vi "Cartesian_to_polar.vi"(2 "Z-Axis (T)":dbl format="%#_13g", 3 "Y-Axis (T)":dbl format="%#_13g") -> (0 "phi (deg)":dbl min=0.0 format="%.3f", 1 "Radial (r) Field (T)":dbl min=0.0 format="%.3f")   [LabVIEW 2018]
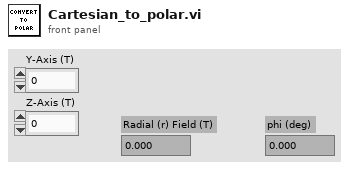
[diagram p1: front panel]
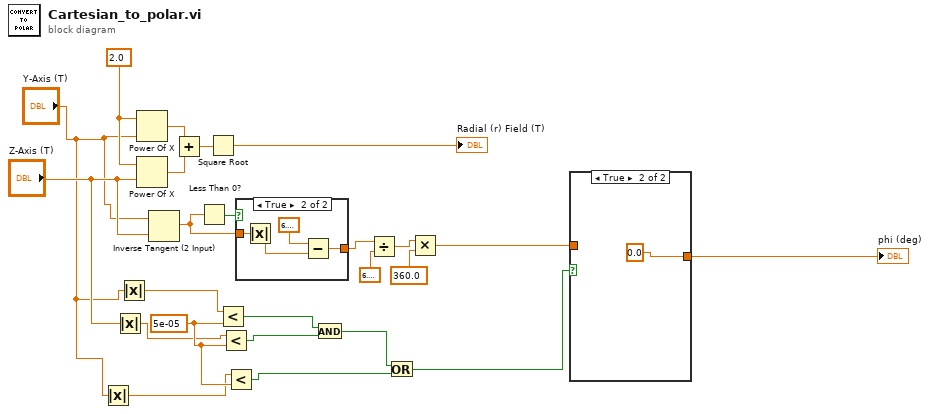
[diagram p0: block diagram]
diagram:
  w7 = 5e-05 ("y")
  w24 = 2.0 ("y")
  n1 = Absolute Value(x="Y-Axis (T)") -> (abs(x)=w5:dbl)
  n2 = Absolute Value(x="Z-Axis (T)") -> (abs(x)=w4:dbl)
  n3 = Absolute Value(x="Y-Axis (T)") -> (abs(x)=w1:dbl)
  n4 = Power Of X(1:"Y-Axis (T)", 2:w24) -> (0:w23:dbl)
  n5 = Power Of X(1:"Z-Axis (T)", 2:w24) -> (0:w22:dbl)
  n6 = Inverse Tangent (2 Input)(1:"Z-Axis (T)", 2:"Y-Axis (T)") -> (0:w19:dbl)
  n7 = Add(x=w23, y=w22) -> (x+y=w21:dbl)
  n8 = Less Than 0?(x=w19) -> (x < 0?=w20:bool)
  n9 = Square Root(x=w21) -> (sqrt(x)=→"Radial (r) Field (T)":dbl)
  n10 = Less?(x=w1, y=w7) -> (x < y?=w12:bool)
  n11 = Less?(x=w4, y=w7) -> (x < y?=w11:bool)
  n12 = Less?(x=w5, y=w7) -> (x < y?=w6:bool)
  n13 = case shown="True" w20 {
    tunnel: w19 -> [w25 w29]
    tunnel: [w25 w27] -> w17
    frame False {
    }
    frame True {
      n14 = Absolute Value(x=w29) -> (abs(x)=w28:dbl)
      n15 = Subtract(x=6.283185307179586, y=w28) -> (x-y=w27:dbl)
    }
  }
  n16 = And(x=w12, y=w11) -> (x .and. y?=w9:bool)
  n17 = Divide(x=w17, y=6.283185307179586) -> (x/y=w14:dbl)
  n18 = Or(x=w9, y=w6) -> (x .or. y?=w8:bool)
  n19 = Multiply(x=w14, y=360.0) -> (x*y=w15:dbl)
  n20 = case shown="True" w8 {
    tunnel: w15 -> [w30 _]
    tunnel: [w30 0.0] -> w10
    frame False {
    }
    frame True {
    }
  }
  "phi (deg)" <- w10
